vi "OnTimeout.vi"(8 "error in (no error)":errorcluster, 10 "Correlation ID":u32, 11 "AutomationContext in":refnum<class "AutomationContext.lvclass">) -> (0 "error out":errorcluster, 3 "AutomationContext out":refnum<class "AutomationContext.lvclass">)   [LabVIEW 2023, in "Automation.lvlib" / "AutomationContext.lvclass"]
uses:
  AutomationContext.lvclass
  AutomationContext.lvclass/AutomationContext.ctl
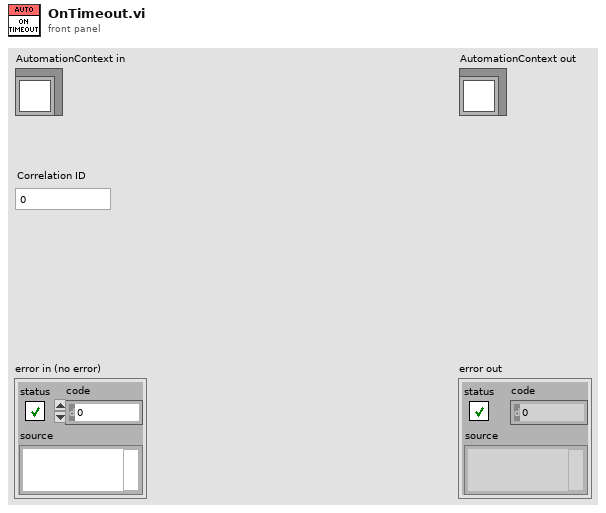
[diagram p1: front panel]
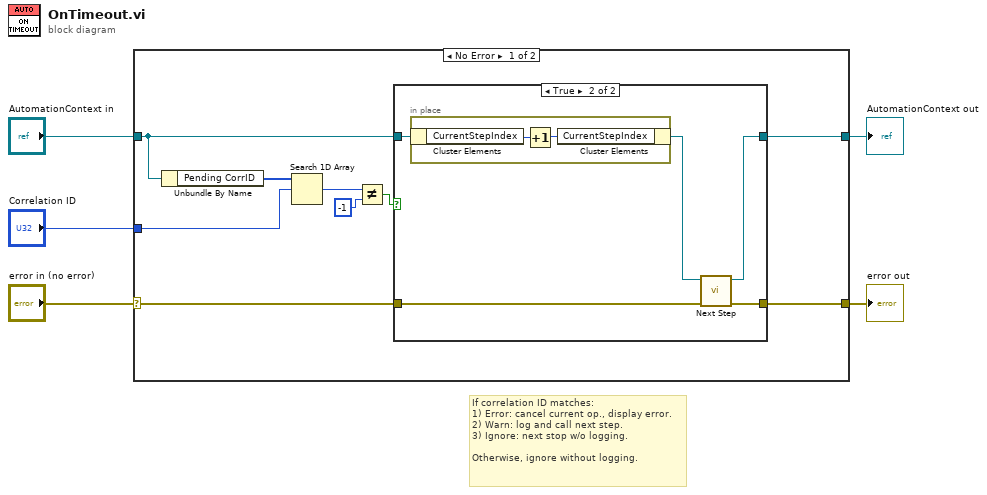
[diagram p0: block diagram]
diagram:
  # "If correlation ID matches:\n1) Error: cancel current op., display error.\n2) Warn: log and call next step.\n3) Ignore: next stop w/o logging.\n\nOtherwise, ignore without logging."
  n1 = case shown="No Error" "error in (no error)" {
    selector: "error in (no error)" -> [w12 w25]
    tunnel: [w11 w25] -> w4
    tunnel: [w13 w24] -> w2
    tunnel: "AutomationContext in" -> [w14 w24]
    tunnel: "Correlation ID" -> [w9 _]
    frame No Error {
      n2 = Unbundle By Name(w14) -> ("Pending CorrID"=w10:u32[])
      n3 = Search 1D Array(1D array=w10, element=w9) -> (index of element=w6:i32)  [unwired: 1 in]
      n4 = Not Equal?(x=w6, y=-1) -> (x != y?=w7:bool)
      n5 = case shown="True" w7 {
        tunnel: w14 -> [w16 w21]
        tunnel: [w16 w17] -> w13
        tunnel: w12 -> [w15 w19]
        tunnel: [w15 w20] -> w11
        frame False {
        }
        frame True {
          n6 = in-place {
            n7 = in-place-cluster #1(w21) -> ("CurrentStepIndex"=w23:u32)
            n8 = Increment(x=w23) -> (x+1=w22:u32)
            n9 = in-place-cluster #1("CurrentStepIndex"=w22) -> (w18:refnum<class "AutomationContext.lvclass">)
          }
          n10 = call "Next Step.vi"("error in (no error)"=w19, "AutomationContext in"=w18) -> ("error out"=w20:errorcluster, "AutomationContext out"=w17:refnum<class "AutomationContext.lvclass">)  [unwired: 8 in]
        }
      }
    }
    frame Error {
    }
  }
  "error out" <- w4
  "AutomationContext out" <- w2
